vi "XLP80_Action_ErrorCodeMessage.vi"(9 "TimeStamp":dbl format="%.2f", 11 "SYS_Error_Code":u32 format="%.0x") -> (3 "message string":string)   [LabVIEW 2021]
uses:
  XLP80_Globals/XLP80_Globals_Status.vi
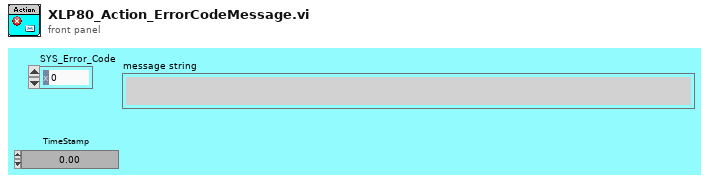
[diagram p1: front panel]
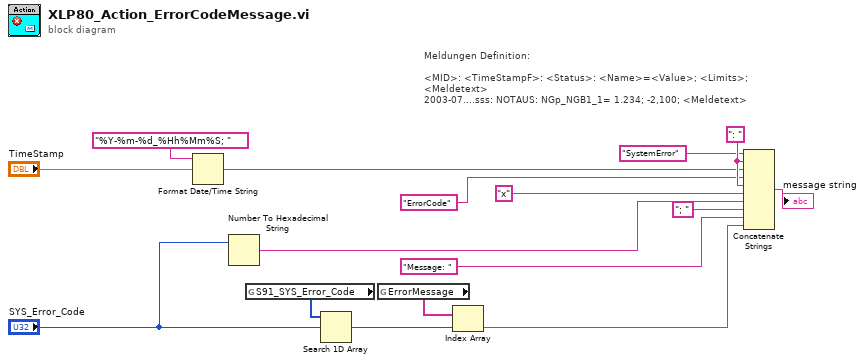
[diagram p0: block diagram]
diagram:
  w16 = ": " ("string")
  # "Meldungen Definition:\n\n<MID>: <TimeStampF>: <Status>: <Name>=<Value>; <Limits>; <Meldetext>\n2003-07....sss: NOTAUS: NGp_NGB1_1= 1.234; -2,100; <Meldetext>"
  n1 = Format Date/Time String(time format string (%c)="%Y-%m-%d_%Hh%Mm%S; ", seconds (now)="TimeStamp") -> (date/time string=w12:string)  [unwired: 1 in]
  n2 = Number To Hexadecimal String(2:"SYS_Error_Code") -> (0:w2:string)  [unwired: 1 in]
  n3 = global read "XLP80_Globals_Status.vi" "S91_SYS_Error_Code"() -> (w8:u32[])
  n4 = Search 1D Array(1D array=w8, element="SYS_Error_Code") -> (index of element=w6:i32)  [unwired: 1 in]
  n5 = global read "XLP80_Globals_Status.vi" "ErrorMessage"() -> (w7:string[])
  n6 = Index Array(array=w7, index=w6) -> (element=w5:string)
  n7 = Concatenate Strings("SystemError" ("string"), w16, w12, "ErrorCode" ("Ring Text.Text"), w16, "x", w2, "; " ("string"), "Message: " ("Ring Text.Text"), w5) -> (→"message string":string)
